vi "Build Depth Arrays.vi"() -> (0 "Array Tiny":u16[](array[numeric]), 1 "Array Low":u16[](array[numeric]))   [LabVIEW 2015]
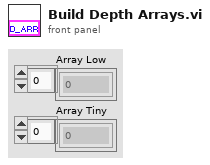
[diagram p1: front panel]
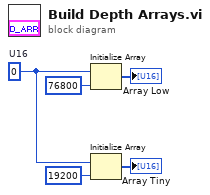
[diagram p0: block diagram]
diagram:
  w5 = u16 0  # U16
  n1 = Initialize Array(w5, 76800 ("dimension size")) -> (→"Array Low":u16[])
  n2 = Initialize Array(w5, 19200 ("dimension size")) -> (→"Array Tiny":u16[])
